vi "Write DM-SetPower-Command-Arguments.vi"(8 "error in (no error)":errorcluster, 10 "DM-SetPower-Command-Initial":T1 {"Power" scale=-1.0..1.0}, 11 "DM-SetPower-Command in":refnum<class "DM-SetPower-Command.lvclass">) -> (0 "error out":errorcluster, 3 "DM-SetPower-Command out":refnum<class "DM-SetPower-Command.lvclass">)   [LabVIEW 2013, in "DM-SetPower-Command.lvclass"]
uses:
  DM-SetPower-Command.lvclass
  DM-SetPower-Command-Arguments.ctl
  DM-SetPower-Command.lvclass/DM-SetPower-Command.ctl
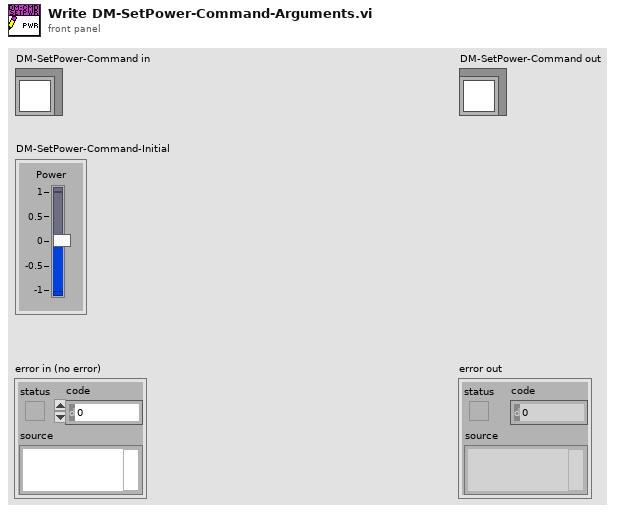
[diagram p1: front panel]
types:
  T1 = typedef "DM-SetPower-Command.lvclass/DM-SetPower-Command-Arguments.ctl" = cluster{"Power":dbl}
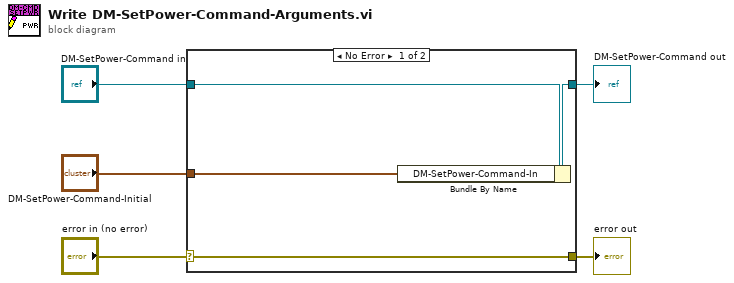
[diagram p0: block diagram]
diagram:
  n1 = case shown="No Error" "error in (no error)" {
    selector: "error in (no error)" -> [w9 w10]
    tunnel: [w9 w10] -> w4
    tunnel: [w7 w11] -> w2
    tunnel: "DM-SetPower-Command in" -> [w8 w11]
    tunnel: "DM-SetPower-Command-Initial" -> [w6 _]
    frame No Error {
      n2 = Bundle By Name(cluster=w8, "DM-SetPower-Command-In"=w6) -> (w7:refnum<class "DM-SetPower-Command.lvclass">)
    }
    frame Error {
    }
  }
  "error out" <- w4
  "DM-SetPower-Command out" <- w2
